vi "9701 Missing Mandatory Sub-Index--error.vi"(8 "error in":errorcluster, 10 "Sub-Index":u16, 11 "Index":u16) -> (0 "error out":errorcluster)   [LabVIEW 2019, in "PDO Grid.lvlib" / "TX PDO Communication Parameter.lvclass"]
uses:
  TX PDO Communication Parameter.lvclass
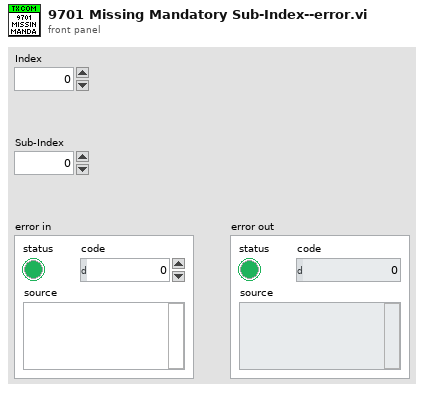
[diagram p1: front panel]
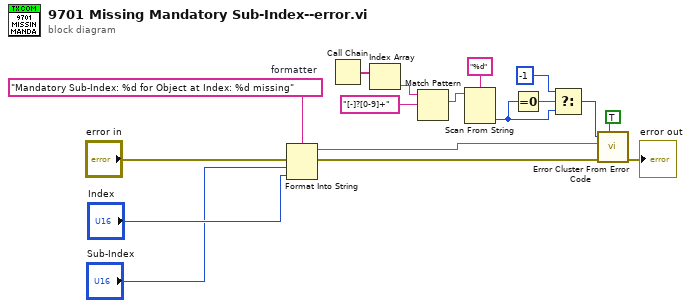
[diagram p0: block diagram]
diagram:
  w14 = "Mandatory Sub-Index: %d for Object at Index: %d missing"  # formatter
  n1 = Format Into String(format string=w14, error in="error in", "Sub-Index", "Index") -> (resulting string=w15:string, error out=w3:errorcluster)  [unwired: 1 in]
  n2 = Call Chain() -> (call chain=w6:string[])
  n3 = Index Array(array=w6) -> (element=w11:string)  [unwired: 1 in]
  n4 = Match Pattern(string=w11, regular expression="[-]?[0-9]+") -> (match substring=w12:string)  [unwired: 1 in, 3 out]
  n5 = Scan From String(format string="%d", input string=w12) -> (output 1=w8:i32)  [unwired: 3 in, 3 out]
  n6 = Equal To 0?(x=w8) -> (x = 0?=w9:bool)
  n7 = Select(t=-1, s=w9, f=w8) -> (s? t:f=w5:i32)
  n8 = call <vilib>:"Error Cluster From Error Code.vi"("show call chain? (False)"=TRUE, "error in (no error)"=w3, "error message (\"\")"=w15, "error code (0)"=w5) -> ("error out"=→"error out":errorcluster)  [unwired: 5 in]
